vi "Override Client Type.vi"(8 "error in (no error)":errorcluster, 11 "TCP Server in":refnum<class "TCP Server.lvclass">) -> (0 "error out":errorcluster, 2 "Override Client Type":refnum<class "TCP Client.lvclass">, 3 "TCP Server out":refnum<class "TCP Server.lvclass">)   [LabVIEW 2024, in "Stream-TCP.lvlib" / "TCP Server.lvclass"]
uses:
  TCP Server.lvclass
  TCP Client/TCP Client.lvclass
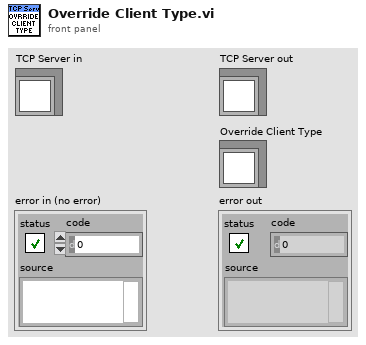
[diagram p1: front panel]
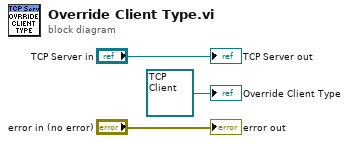
[diagram p0: block diagram]
diagram:
  "error out" <- "error in (no error)"
  "TCP Server out" <- "TCP Server in"
  "Override Client Type" <- refnum<class "TCP Client.lvclass"> refnum ("Stream-TCP:TCP Client")
